vi "AddFailureReference.vi"(8 "error in":errorcluster, 10 "Id":string, 11 "SequenceRun in":refnum<class "SequenceRun.lvclass">) -> (0 "error out":errorcluster, 2 "Document":refnum<class "FailureReference.lvclass">, 3 "SequenceRun out":refnum<class "SequenceRun.lvclass">)   [LabVIEW 2021, in "ProligentXMLGenerator.lvlib" / "SequenceRun.lvclass"]
doc: "Add a StepRun.\n\nA step run is a time-bound logical container for a set of measures.\nA step run is uniquely identified by its StepRunId."
uses:
  SequenceRun.lvclass
  SequenceRun.lvclass/SequenceRun.ctl
  Failure/FailureReference/FailureReference.lvclass
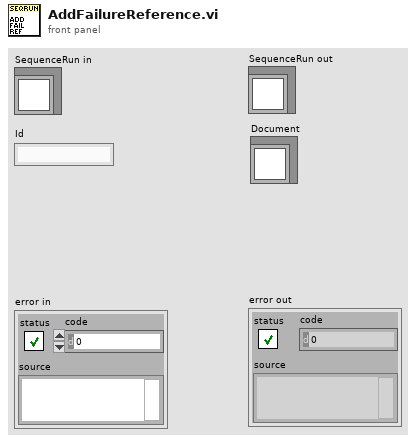
[diagram p1: front panel]
types:
  T1 = typedef "ProligentXMLGenerator.lvlib/SequenceRun.lvclass/Data.ctl" = cluster{"Name":string, "StepRuns":refnum<class "StepRun.lvclass">[], "Characteristics":refnum<class "Characteristic.lvclass">[], "Documents":refnum<class "Document.lvclass">[], "FailureReferences":refnum<class "FailureReference.lvclass">[], "CustomData":refnum<class "CustomData.lvclass">, "StartDate":refnum<class "DateTime.lvclass">, "EndDate":refnum<class "DateTime.lvclass">, "SequenceExecutionStatus":refnum<class "ExecutionStatus.lvclass">, "SequenceRunId":refnum<class "Guid.lvclass">, "SequenceFullName":refnum<class "SequenceFullName.lvclass">, "SequenceVersion":refnum<class "NonEmptyString_64.lvclass">, "StationFullName":refnum<class "FullName.lvclass">, "User":refnum<class "NonEmptyString_255.lvclass">, "TimeZoneInfoId":string}
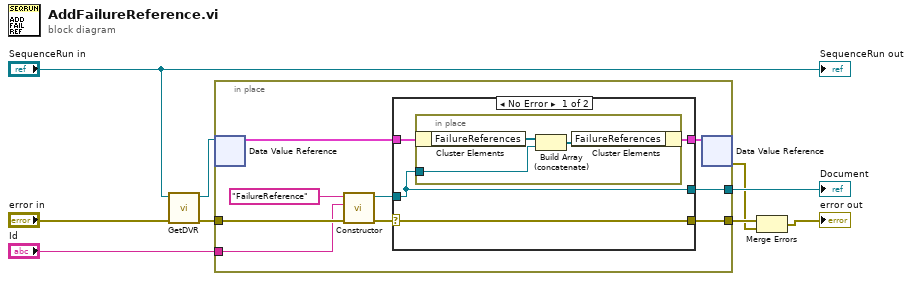
[diagram p0: block diagram]
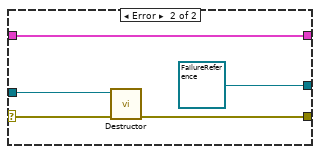
[diagram p2: hidden frame]
diagram:
  n1 = call "GetDVR.vi"("error in"="error in", "SequenceRun"="SequenceRun in") -> ("error out"=w3:errorcluster, "DVRReference"=w2:refnum<data-value>)  [unwired: 8 in]
  n2 = in-place "In Place Element Structure" {
    in-place-border: "Id" -> [w10]
    in-place-border: [w17] -> w4
    in-place-border: w3 -> [w16]
    in-place-border: [w13] -> w5
    n3 = in-place-dvr #1(w2) -> (w15:T1)  [unwired: 1 out]
    n4 = call "Constructor.vi"("error in"=w16, "Id"=w10, "Name"="FailureReference") -> ("error out"=w18:errorcluster, "FailureReference out"=w12:refnum<class "FailureReference.lvclass">)  [unwired: 7 in]
    n5 = case shown="No Error" w18 {
      selector: w18 -> [w22 w29]
      tunnel: [w19 w30] -> w14
      tunnel: [w22 w28] -> w17
      tunnel: w12 -> [w21 w27]
      tunnel: w15 -> [w20 w30]
      tunnel: [w21 refnum<class "FailureReference.lvclass"> refnum ("ProligentResultProcessor:FailureReference")] -> w13
      frame No Error {
        n6 = in-place "In Place Element Structure" {
          in-place-border: w21 -> [w25]
          n7 = in-place-cluster #2(w20) -> ("FailureReferences"=w24:refnum<class "FailureReference.lvclass">[])
          n8 = Build Array (concatenate)(w24, w25) -> (w23:refnum<class "FailureReference.lvclass">[])
          n9 = in-place-cluster #2("FailureReferences"=w23) -> (w19:T1)
        }
      }
      frame Error {
        n10 = call "Destructor.vi"("error in"=w29, "FailureReference in"=w27) -> ("error out"=w28:errorcluster)  [unwired: 9 in]
      }
    }
    n11 = in-place-dvr #1(w14) -> (w1:errorcluster)  [unwired: 1 out]
  }
  "Document" <- w5
  n12 = Merge Errors(w4, w1) -> (→"error out":errorcluster)
  "SequenceRun out" <- "SequenceRun in"
